vi "Read Header Column size and Table size.vi"(0 "Pdfp Table Class in":refnum<class "Pdfp Table Class.lvclass">, 11 "error in (no error)":errorcluster) -> (4 "Pdfp Table Class out":refnum<class "Pdfp Table Class.lvclass">, 6 "Header Column size":cluster{"# Column":u16, "# Row":u16}, 8 "Table size":cluster{"# Column":u16, "# Row":u16}, 10 "Row Header?":bool, 15 "error out":errorcluster)   [LabVIEW 2019, in "Pdfp Table Class.lvclass"]
uses:
  <userlib>/Exaprom PDF/LV Class/Pdfp Table Class/Pdfp Table Class.lvclass
  <userlib>/Exaprom PDF/LV Class/Pdfp Table Class/Pdfp Table Class.lvclass/Pdfp Table Class.ctl
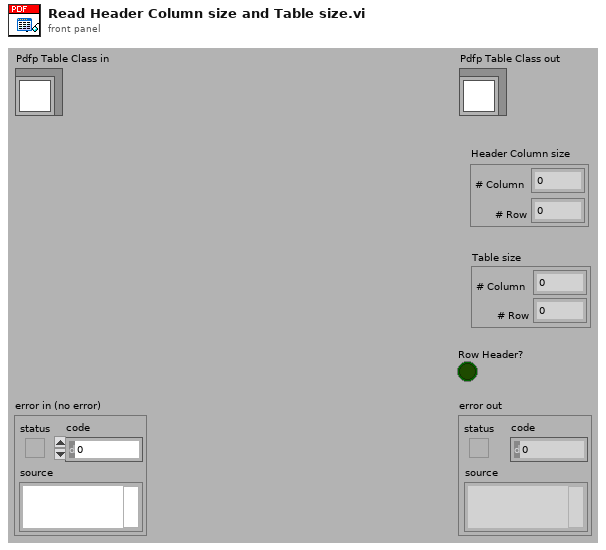
[diagram p1: front panel]
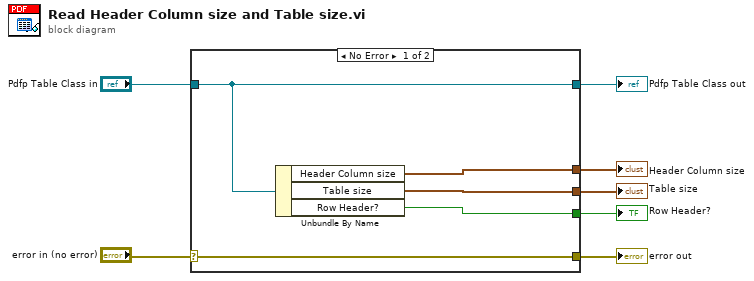
[diagram p0: block diagram]
diagram:
  n1 = case shown="No Error" "error in (no error)" {
    selector: "error in (no error)" -> [w12 w13]
    tunnel: [w12 w13] -> w6
    tunnel: [w11 w14] -> w4
    tunnel: "Pdfp Table Class in" -> [w11 w14]
    tunnel: [w10 _] -> w3
    tunnel: [w9 _] -> w2
    tunnel: [w8 _] -> w1
    frame No Error {
      n2 = Unbundle By Name(w11) -> ("Header Column size"=w10:cluster{"# Column":u16, "# Row":u16}, "Table size"=w9:cluster{"# Column":u16, "# Row":u16}, "Row Header?"=w8:bool)
    }
    frame Error {
    }
  }
  "error out" <- w6
  "Pdfp Table Class out" <- w4
  "Header Column size" <- w3
  "Table size" <- w2
  "Row Header?" <- w1
